vi "Deadband.vi"(8 "+- Bounds":dbl=0.3 format="%#_13g", 11 "Raw Value":dbl format="%#_13g") -> (2 "Filtered Value":dbl format="%#_13g")   [LabVIEW 2017]
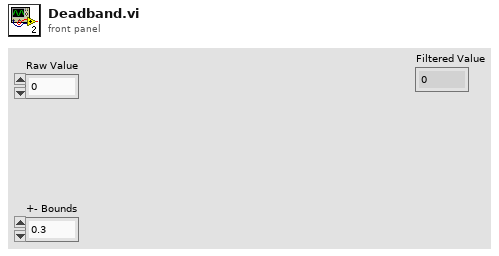
[diagram p1: front panel]
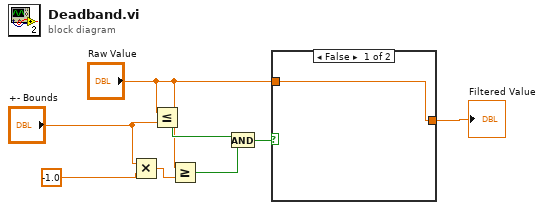
[diagram p0: block diagram]
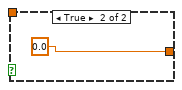
[diagram p2: hidden frame]
diagram:
  n1 = Multiply(x="+- Bounds", y=-1.0 ("Numeric")) -> (x*y=w6:dbl)
  n2 = Less Or Equal?(x="Raw Value", y="+- Bounds") -> (x <= y?=w3:bool)
  n3 = Greater Or Equal?(x="Raw Value", y=w6) -> (x >= y?=w5:bool)
  n4 = And(x=w3, y=w5) -> (x .and. y?=w4:bool)
  n5 = case shown="False" w4 {
    tunnel: [w9 0.0 ("Y axis value")] -> w2
    tunnel: "Raw Value" -> [w9 _]
    frame False {
    }
    frame True {
    }
  }
  "Filtered Value" <- w2
